vi "Server System Main.vi"   [LabVIEW 2020, in "VolatusScratch.lvlib" / "StandaloneServer.lvlib"]
uses:
  StandaloneServer.lvlib
  Volatus/Volatus Core/Volatus Core.lvclass
  Volatus/Volatus.lvlib
  Volatus/MessageQ/MessageQ.lvclass
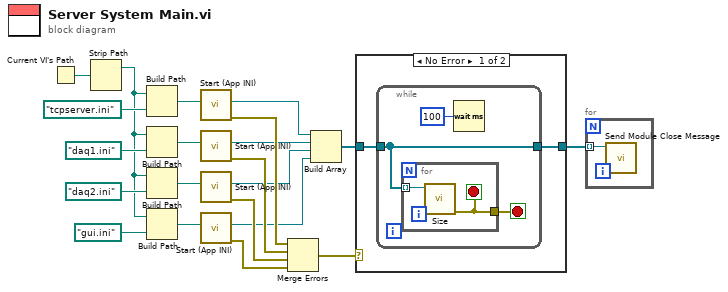
[diagram p0: block diagram]
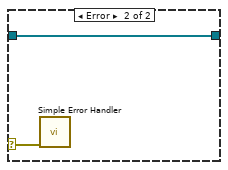
[diagram p2: hidden frame]
diagram:
  n1 = Current VI's Path() -> (path=w20:path)
  n2 = Strip Path(path=w20) -> (stripped path=w16:path)  [unwired: 1 out]
  n3 = Build Path(base path=w16, name or relative path=path "tcpserver.ini") -> (appended path=w15:path)
  n4 = Build Path(base path=w16, name or relative path=path "daq1.ini") -> (appended path=w14:path)
  n5 = Build Path(base path=w16, name or relative path=path "daq2.ini") -> (appended path=w13:path)
  n6 = Build Path(base path=w16, name or relative path=path "gui.ini") -> (appended path=w12:path)
  n7 = call "Start (App INI).vi"("INI Path (Default)"=w15) -> ("error out"=w11:errorcluster, "MessageQ"=w5:refnum<class "MessageQ.lvclass">)  [unwired: 9 in]
  n8 = call "Start (App INI).vi"("INI Path (Default)"=w14) -> ("error out"=w10:errorcluster, "MessageQ"=w6:refnum<class "MessageQ.lvclass">)  [unwired: 9 in]
  n9 = call "Start (App INI).vi"("INI Path (Default)"=w13) -> ("error out"=w9:errorcluster, "MessageQ"=w4:refnum<class "MessageQ.lvclass">)  [unwired: 9 in]
  n10 = call "Start (App INI).vi"("INI Path (Default)"=w12) -> ("error out"=w8:errorcluster, "MessageQ"=w3:refnum<class "MessageQ.lvclass">)  [unwired: 9 in]
  n11 = Merge Errors(w11, w10, w9, w8) -> (w7:errorcluster)
  n12 = Build Array(w5, w6, w4, w3) -> (w2:refnum<class "MessageQ.lvclass">[])
  n13 = case shown="No Error" w7 {
    selector: w7 -> [_ w30]
    tunnel: w2 -> [w23 w29]
    tunnel: [w22 w29] -> w1
    frame No Error {
      n14 = while {
        tunnel: w23 -> [w25]
        tunnel: [w25] -> w22
        stop <- w26 stop-if-true
        n15 = for {
          tunnel: [w28] -> w26
          tunnel: w25 -> [w27] mode=indexing
          stop <- w28 stop-if-true
          n16 = call "Size.vi"("MessageQ in"=w27) -> ("error out"=w28:errorcluster)  [unwired: 7 in, 3 out]
        }
        n17 = Wait (ms)(milliseconds to wait=u32 100) -> ()  [unwired: 1 out]
      }
    }
    frame Error {
      n18 = call <vilib>:"Simple Error Handler.vi"("error in (no error)"=w30) -> ()  [unwired: 4 in, 5 out]
    }
  }
  n19 = for {
    tunnel: w1 -> [w31] mode=indexing
    n20 = call "Send Module Close Message.vi"("MessageQ"=w31) -> ()  [unwired: 10 in, 1 out]
  }
